vi "Read_Write_VCNL4010.vi"(8 "error in (no error)":errorcluster, 10 "i_Ref":T2, 11 "Register Adress":u8) -> (0 "error out":errorcluster, 3 "Bytes Read":u8[](array[numeric]))   [LabVIEW 2016]
panel:
  in  "i_Ref 2":T1={"Adress"=19, "CMD"=enum."#0 V_Sensor", "i_Value"=0, "R/W"=enum."Read"} {"i_Value" format="%.0b"; "Adress" format="%02x"}
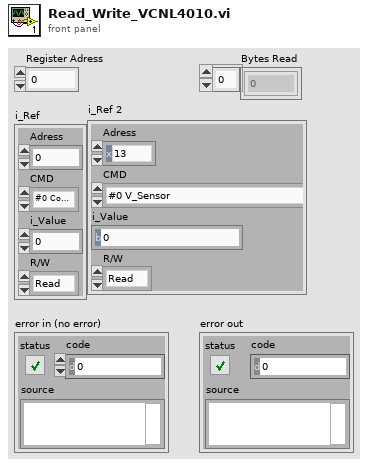
[diagram p1: front panel]
types:
  T1 = cluster{"Adress":u8, "CMD":enum8{"#0 V_Sensor", "#1 T_Die", "#2 Configuration", "#3 T_Obj", "#4 Status", "#5 Status mask and enable", "#6 T_Obj high limit", "#7 T_Obj low-limit", "#8 T_Die high-limit", "#9 T_Die low-limit", "#0A S0 coefficient ", "#0B A1 Coefficient", "#0C A2 Coefficient", "#0D B0 Coefficient", "#0E B1 Coefficient", "#0F B2Coefficient", "#10 C2 Coefficient", "#11 TC0 Coefficientd", "#12 TC1 Coefficient", "#1E Manufacturer ID", "#1F Device ID", "#2A Memory access"}, "i_Value":u16, "R/W":enum16{"Read", "Write"}}
  T2 = cluster{"Adress":u8, "CMD":enum8{"#0 Command Register", "#1 Product ID Revision Register", "#2 Proximity Rate Register", "#3 IR LED Current Register", "#4 Ambient Light Parameter Register", "#5 Ambient Light Result Register", "#6 Ambient Light Result Register", "#7 Proximity Result Register", "#8 Proximity Result Register", "#9 Interrupt Control Register", "#10 Low Threshold Register", "#11 Low Threshold Register", "#12 High Threshold Register", "#13 High Threshold Register", "#14 Interrupt Status Register", "#15 Proximity Modulation Timing Adjustment"}, "i_Value":u8, "R/W":enum16{"Read", "Write"}}
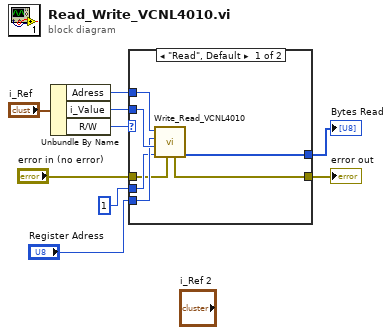
[diagram p0: block diagram]
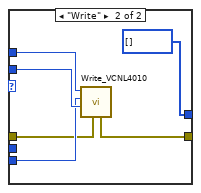
[diagram p2: hidden frame]
diagram:
  n1 = Unbundle By Name("i_Ref") -> ("Adress"=w3:u8, "i_Value"=w4:u8, "R/W"=w2:enum16{"Read", "Write"})
  n2 = case shown="\"Read\", Default" w2 {
    tunnel: [w16 w22] -> w9
    tunnel: [w15 u8[] [] ("Bytes Read")] -> w8
    tunnel: w3 -> [w14 w20]
    tunnel: w4 -> [w13 w19]
    tunnel: "Register Adress" -> [w12 w18]
    tunnel: u32 1 ("Byte Count") -> [w11 _]
    tunnel: "error in (no error)" -> [w10 w17]
    frame "Read", Default {
      n3 = call "Write_Read_VCNL4010.vi"("i_error"=w10, "Byte Count"=w11, "i_Data byte"=w13, "Register Adress"=w12, "Slave Adress"=w14) -> ("Bytes Read"=w15:u8[], "o_error"=w16:errorcluster)  [unwired: 5 in]
    }
    frame "Write" {
      n4 = call "Write_VCNL4010.vi"("i_error"=w17, "i_Data byte"=w19, "Register Adress"=w18, "Slave Adress"=w20) -> ("o_error"=w22:errorcluster)  [unwired: 7 in]
    }
  }
  "error out" <- w9
  "Bytes Read" <- w8
